vi "Tosca-Retrieve Final Event Times.vi"(0 "IP Address":string, 5 "Port":i32, 11 "error in (no error)":errorcluster) -> (4 "Codes":i16[](array[numeric]), 8 "Times":sgl[](array[numeric]), 15 "error out":errorcluster)   [LabVIEW 2020]
panel:
  # "Retrieving final data from Synapse..."
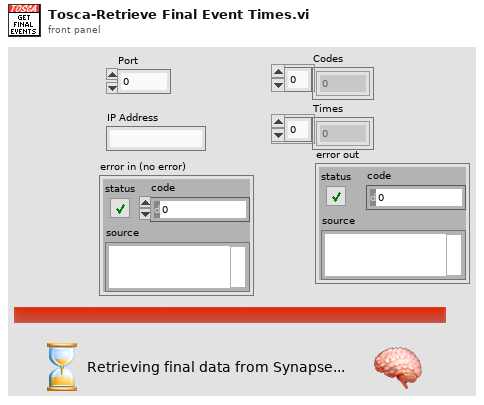
[diagram p1: front panel]
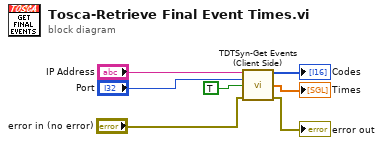
[diagram p0: block diagram]
diagram:
  n1 = call "TDTSyn-Get Events (Client Side).vi"("IP Address"="IP Address", "Port"="Port", "last read"=TRUE, "error in (no error)"="error in (no error)") -> ("Codes"=→"Codes":i16[], "Times"=→"Times":sgl[], "error out"=→"error out":errorcluster)  [unwired: 9 in]
